vi "ex4-8.vi"() -> ()   [LabVIEW 2009]
uses:
  <vilib>/NXT/Dual Mode Library/Waits/Wait_Num.vi
  <vilib>/NXT/Dual Mode Library/Motors/MotorOn.vi
panel:
  in  "Numeric":dbl
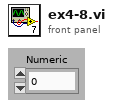
[diagram p1: front panel]
types:
  T1 = typedef "LVHSConnector.ctl" = cluster{"error":errorcluster, "address":string, "NXT #":i32, "Show Error":bool, "Connection":u16}
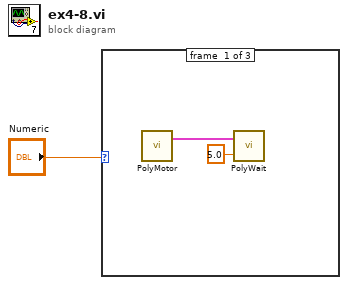
[diagram p0: block diagram]
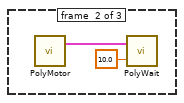
[diagram p2: hidden frame]
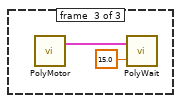
[diagram p3: hidden frame]
diagram:
  n1 = case shown="1, Default" "Numeric" {
    frame #0 {
      n2 = call-poly <vilib>:"PolyMotor.vi"() -> ("NXT"=w3:T1)  [unwired: 4 in]
      n3 = call-poly <vilib>:"PolyWait.vi"("Time (1 sec)"=sgl 5.0, "NXT"=w3) -> ()  [unwired: 2 in, 1 out]
    }
    frame #1 {
      n4 = call-poly <vilib>:"PolyMotor.vi"() -> ("NXT"=w4:T1)  [unwired: 4 in]
      n5 = call-poly <vilib>:"PolyWait.vi"("Time (1 sec)"=sgl 10.0, "NXT"=w4) -> ()  [unwired: 2 in, 1 out]
    }
    frame #2 {
      n6 = call-poly <vilib>:"PolyMotor.vi"() -> ("NXT"=w6:T1)  [unwired: 4 in]
      n7 = call-poly <vilib>:"PolyWait.vi"("Time (1 sec)"=sgl 15.0, "NXT"=w6) -> ()  [unwired: 2 in, 1 out]
    }
  }
